vi "Pre Launch Init.vi"(11 "Simulated Entry Console in":refnum<class "Simulated Entry Console.lvclass">) -> (0 "error out":errorcluster, 3 "Simulated Entry Console out":refnum<class "Simulated Entry Console.lvclass">)   [LabVIEW 2012, in "Simulated Entry Console.lvlib" / "Simulated Entry Console.lvclass"]
doc: "(<B>Filename</B>: Actor Framework.lvlib:Actor.lvclass:Pre Launch Init.vi)\n\nDefines behavior that occurs after the Launch Actor method is invoked but before the actor's Actor Core method begins running.\n\nThe Pre Launch Init method is guaranteed to finish before the Launch Actor method returns to its caller and before the actor itself receives any messages. Any references that the Pre Launch Init method obtains are guaranteed to have the same lifetime as the actor itself. Any errors that the Pre Launch Init method returns will abort the launch.\n\nBy default, this method does nothing. A descendant class may override it to define behavior."
uses:
  Simulated Entry Console.lvclass
  Entry Console API/Entry Console API/Entry Console API.lvclass
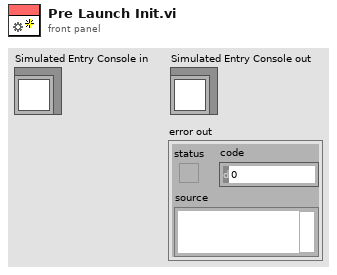
[diagram p1: front panel]
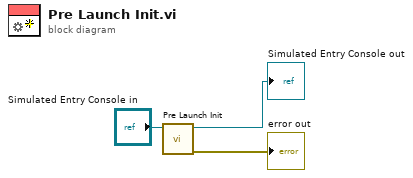
[diagram p0: block diagram]
diagram:
  n1 = call-parent "Pre Launch Init.vi"("Actor in"="Simulated Entry Console in") -> ("error out"=→"error out":errorcluster, "Actor out"=→"Simulated Entry Console out":refnum<class "Simulated Entry Console.lvclass">)  [unwired: 9 in]
